vi "Initialize.vi"(6 "Start Direction":T1=enum."E", 8 "error in (no error)":errorcluster, 9 "Kamikaze DVR":T2, 10 "SquareStatus DVR":T3, 11 "Mother in":refnum<class "Formics.lvclass">) -> (0 "error out":errorcluster, 3 "Mother out":refnum<class "Formics.lvclass">)   [LabVIEW 2015, in "Formics.lvclass"]
uses:
  Formics.lvclass
  SquareStatus DVR.ctl
  Kamikaze DVR.ctl
  Type Defs/Direction Enum.ctl
  Action Queue Element.ctl
  Type Defs/Action Enum.ctl
  Formics.lvclass/Formics.ctl
  Type Defs/SB Type Defs.lvlib
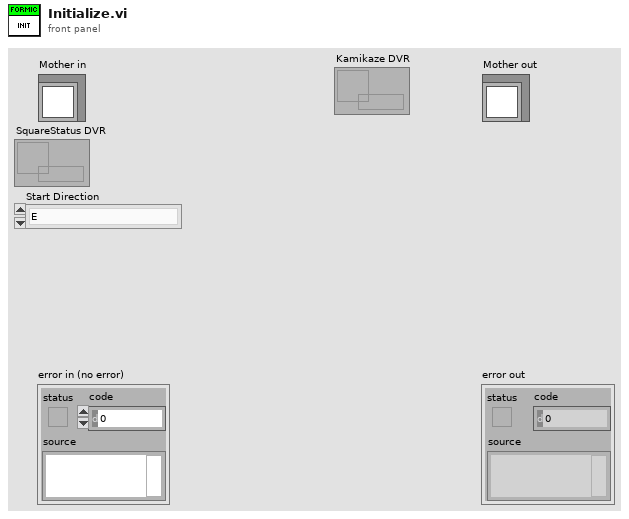
[diagram p1: front panel]
types:
  T1 = typedef "SB Type Defs.lvlib/Direction Enum.ctl" = enum16{"NW", "N", "NE", "E", "SE", "S", "SW", "W"}
  T2 = typedef "Formics.lvclass/Kamikaze DVR.ctl" = refnum<data-value>
  T3 = typedef "Formics.lvclass/SquareStatus DVR.ctl" = refnum<data-value>
  T4 = typedef "Formics.lvclass/Action Queue Element.ctl" = cluster{"Action":T5, "Times":i32}
  T5 = typedef "SB Type Defs.lvlib/Action Enum.ctl" = enum16{"Wait", "Move", "Attack", "Replicate"}
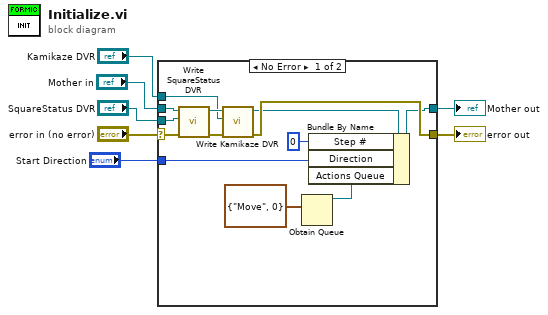
[diagram p0: block diagram]
diagram:
  n1 = case shown="No Error" "error in (no error)" {
    selector: "error in (no error)" -> [w20 w22]
    tunnel: [w14 w22] -> w6
    tunnel: [w12 w21] -> w4
    tunnel: "Mother in" -> [w18 w21]
    tunnel: "SquareStatus DVR" -> [w17 _]
    tunnel: "Kamikaze DVR" -> [w15 _]
    tunnel: "Start Direction" -> [w11 _]
    frame No Error {
      n2 = call-dynamic "Write SquareStatus DVR.vi"("error in (no error)"=w20, "data value reference"=w17, "Mother in"=w18) -> ("error out"=w19:errorcluster, "Mother out"=w16:refnum<class "Formics.lvclass">)  [unwired: 7 in]
      n3 = call "Write Kamikaze DVR.vi"("error in (no error)"=w19, "Kamikaze DVR"=w15, "Mother in"=w16) -> ("error out"=w14:errorcluster, "Mother out"=w13:refnum<class "Formics.lvclass">)  [unwired: 7 in]
      n4 = Obtain Queue(element data type=T4 {"Action"=enum."Move", "Times"=0}) -> (queue out=w9:refnum<queue>)  [unwired: 4 in, 2 out]
      n5 = Bundle By Name(cluster=w13, "Step #"=0, "Direction"=w11, "Actions Queue"=w9) -> (w12:refnum<class "Formics.lvclass">)
    }
    frame Error {
    }
  }
  "error out" <- w6
  "Mother out" <- w4
